vi "Init Drive Motors.vi"   [LabVIEW 2016]
uses:
  <vilib>/Rock Robotics/WPI/ThirdParty/CanMotor/TalonSRX/WPI_CANTalonSRX_APIControlMode.ctl
  <vilib>/Rock Robotics/WPI/RobotDrive/WPI_RobotDriveOpen4MotorWithExistingMotors.vi
  <vilib>/Rock Robotics/WPI/RobotDrive/WPI_RobotDriveOpen2MotorWithExistingMotors.vi
types:
  T1 = typedef "WPI_CANTalonSRX_APIControlMode.ctl" = enum8{"Percent VBus", "Speed", "Position", "Slave", "Unchanged / Invalid", "Voltage Compensation", "Current", "Motion Profile", "Motion Magic"}
  T2 = typedef "WPI_MotorControlDeviceRef.ctl" = cluster{"DeviceStatus":errorcluster, "Type":T3, "PWM":cluster{"PWM Channel":T4, "DeadBand":T5}, "CAN":cluster{"Device Number":u8, "SetOutput VI Ref":variant, "GetOutput VI Ref":variant, "Enable VI Ref":variant, "Disable VI Ref":variant, "Data":variant}, "Invert":bool}
  T3 = typedef "WPI_MotorControlType.ctl" = enum16{"PWM", "CAN"}
  T4 = typedef "FPGA_DIOPWMChannel.ctl" = enum8{"PWM 0", "PWM 1", "PWM 2", "PWM 3", "PWM 4", "PWM 5", "PWM 6", "PWM 7", "PWM 8", "PWM 9", "PWM MXP 0", "PWM MXP 1", "PWM MXP 2", "PWM MXP 3", "PWM MXP 4", "PWM MXP 5", "PWM MXP 6", "PWM MXP 7", "PWM MXP 8", "PWM MXP 9", "Invalid"}
  T5 = typedef "WPI_PWMDeadband.ctl" = cluster{"Name":string, "maxPositivePwm":i32, "minPositivePwm":i32, "centerPwm":i32, "maxNegativePwm":i32, "minNegativePwm":i32, "angularRange":u16}
  T6 = typedef "WPI_RobotDriveDevRef.ctl" = cluster{"DevStatus":errorcluster, "Motors[]":T2[], "Square Inputs":bool, "Max Output":dbl}
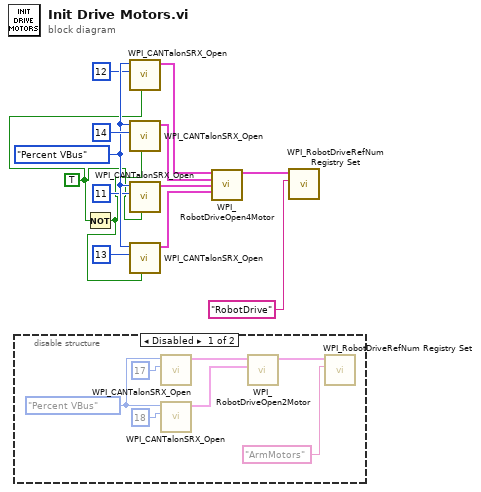
[diagram p0: block diagram]
diagram:
  w2 = TRUE ("Invert")
  w11 = WPI_CANTalonSRX_APIControlMode."Percent VBus" ("Control Mode")
  n1 = disable-structure shown="Disabled" {
    frame Disabled {
      w20 = WPI_CANTalonSRX_APIControlMode."Percent VBus" ("Control Mode")
      n2 = call <vilib>:"WPI_CANTalonSRX_Open.vi"("Device Number"=u8 17, "Control Mode"=w20) -> ("CAN Talon SRX Ref"=w17:T2)  [unwired: 8 in, 1 out]
      n3 = call <vilib>:"WPI_CANTalonSRX_Open.vi"("Device Number"=u8 18, "Control Mode"=w20) -> ("CAN Talon SRX Ref"=w16:T2)  [unwired: 8 in, 1 out]
      n4 = call-poly <vilib>:"WPI_RobotDriveOpen2Motor.vi"("Right Motor Dev Ref"=w16, "Left Motor Dev Ref"=w17) -> ("RobotDriveDevRef"=w15:T6)  [unwired: 8 in, 1 out]
      n5 = call <vilib>:"WPI_RobotDriveRefNum Registry Set.vi"("refnum name"="ArmMotors", "RobotDriveDevRef"=w15) -> ()  [unwired: 8 in, 2 out]
    }
    frame Enabled {
    }
  }
  n6 = Not(x=w2) -> (.not. x?=w1:bool)
  n7 = call <vilib>:"WPI_CANTalonSRX_Open.vi"("Invert"=w2, "Device Number"=u8 12, "Control Mode"=w11) -> ("CAN Talon SRX Ref"=w6:T2)  [unwired: 7 in, 1 out]
  n8 = call <vilib>:"WPI_CANTalonSRX_Open.vi"("Invert"=w1, "Device Number"=u8 14, "Control Mode"=w11) -> ("CAN Talon SRX Ref"=w5:T2)  [unwired: 7 in, 1 out]
  n9 = call <vilib>:"WPI_CANTalonSRX_Open.vi"("Invert"=w2, "Device Number"=u8 11, "Control Mode"=w11) -> ("CAN Talon SRX Ref"=w4:T2)  [unwired: 7 in, 1 out]
  n10 = call <vilib>:"WPI_CANTalonSRX_Open.vi"("Invert"=w1, "Device Number"=u8 13, "Control Mode"=w11) -> ("CAN Talon SRX Ref"=w3:T2)  [unwired: 7 in, 1 out]
  n11 = call-poly <vilib>:"WPI_RobotDriveOpen4Motor.vi"("Rear Left Motor Dev Ref"=w6, "Rear Right Motor Dev Ref"=w5, "Front Left Motor Dev Ref"=w4, "Front Right Motor Dev Ref"=w3) -> ("RobotDriveDevRef"=w8:T6)  [unwired: 10 in, 1 out]
  n12 = call <vilib>:"WPI_RobotDriveRefNum Registry Set.vi"("refnum name"="RobotDrive", "RobotDriveDevRef"=w8) -> ()  [unwired: 8 in, 2 out]
